vi "Item Filter.vi"(6 "Answer":T2, 10 "Item":string, 11 "Classfy In":T1[](array[typedef])) -> (3 "Classfy Out":T1[](array[typedef]))   [LabVIEW 2018]
uses:
  Data Def/Classify.ctl
  Data Def/Answer.ctl
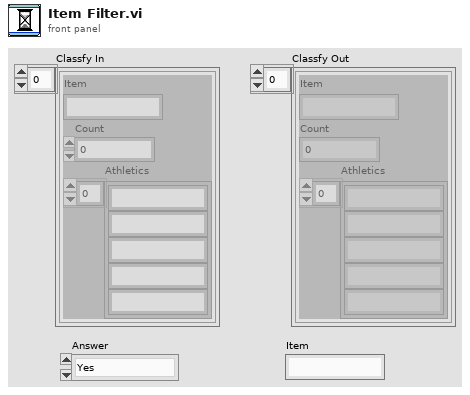
[diagram p1: front panel]
types:
  T1 = typedef "Classify.ctl" = cluster{"Item":string, "Count":i32, "Athletics":string[]}
  T2 = typedef "Answer.ctl" = enum16{"Yes", "No", "I don't Know"}
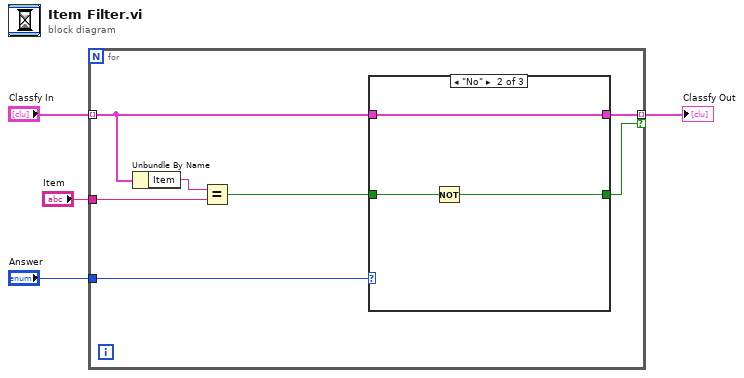
[diagram p0: block diagram]
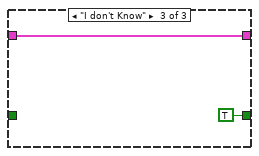
[diagram p3: hidden frame]
diagram:
  n1 = for {
    tunnel: "Classfy In" -> [w11] mode=indexing
    tunnel: [w10] -> w4 mode=indexing if=w8
    tunnel: "Answer" -> [w9]
    tunnel: "Item" -> [w6]
    n2 = Unbundle By Name(w11) -> ("Item"=w7:string)
    n3 = Equal?(x=w7, y=w6) -> (x = y?=w5:bool)
    n4 = case shown="\"No\"" w9 {
      tunnel: w11 -> [w13 w16 w18]
      tunnel: [w13 w16 w18] -> w10
      tunnel: [w12 w15 TRUE] -> w8
      tunnel: w5 -> [w12 w14 _]
      frame "Yes", Default {
      }
      frame "No" {
        n5 = Not(x=w14) -> (.not. x?=w15:bool)
      }
      frame "I don't Know" {
      }
    }
  }
  "Classfy Out" <- w4
